vi "LaunchPad Logging Loop.vi"(11 "Queue in":refnum<queue>) -> ()   [LabVIEW 2015]
uses:
  Telemetry Packet Type.ctl
  Thermocouple Data.ctl
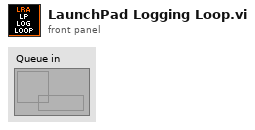
[diagram p1: front panel]
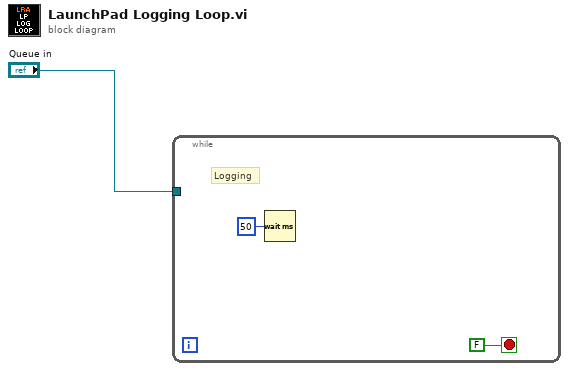
[diagram p0: block diagram]
diagram:
  n1 = while {
    tunnel: "Queue in" -> [_]
    stop <- FALSE stop-if-true
    # "Logging"
    n2 = Wait (ms)(milliseconds to wait=u32 50) -> ()  [unwired: 1 out]
  }
